vi "DSF.Engine.Plugin.Get Cache.vi"(11 "Plugin in":refnum<class "DSF.Engine.Plugin.lvclass">) -> (2 "Cache":refnum<class "DSF.Engine.Memory.Cache.lvclass">, 3 "Plugin out":refnum<class "DSF.Engine.Plugin.lvclass">)   [LabVIEW 2017, in "DSF.Engine.lvlib" / "DSF.Engine.Plugin.lvclass"]
uses:
  DSF.Engine.Plugin.lvclass
  Cache/DSF.Engine.Memory.Cache.lvclass
  DSF.Engine.Plugin.lvclass/DSF.Engine.Plugin.ctl
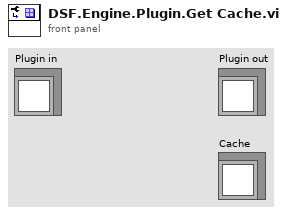
[diagram p1: front panel]
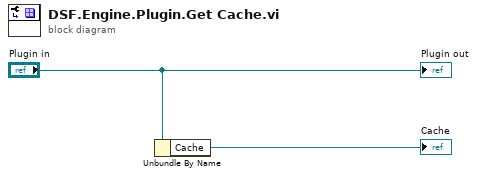
[diagram p0: block diagram]
diagram:
  n1 = Unbundle By Name("Plugin in") -> ("Cache"=→"Cache":refnum<class "DSF.Engine.Memory.Cache.lvclass">)
  "Plugin out" <- "Plugin in"
